vi "getHWIO_4_statusExpos.vi"(0 "Camera in":refnum<class "Camera.lvclass">, 5 "error in (no error)":errorcluster) -> (14 "Camera out":refnum<class "Camera.lvclass">, 15 "on":bool=TRUE, 16 "polarity":u16(ring)=1 items=["high level"=1, "low level"=2], 17 "signal_type":u32(ring)=1 items=["Status Busy", "Status Expos", "Status Line", "Status Armed"], 18 "signal_timing":u32(ring) items=["undefined", "first line", "global", "last line", "all lines"], 19 "error out":errorcluster)   [LabVIEW 2019, in "Camera.lvclass"]
doc: "Gets polarity, status (enabled / disabled), fuction (exposure or line) and signal timing (first line, last line, all lines, global) for the HWIO 4 status expose signal. Generates an error if camera is recording or if HWIO configuration is not supported. Signal timing is ignored if the signal function is not Status Expose."
uses:
  Camera.lvclass
  pco.sdk/TimingControl/TimingControl.lvlib
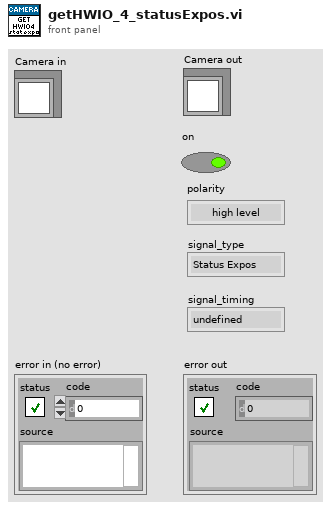
[diagram p1: front panel]
types:
  T1 = cluster{"wSignalNum":u16, "wEnabled":u16, "wType":u16, "wPolarity":u16, "wFilterSetting":u16, "wSelected":u16, "dwParameter":u32[], "dwSignalFunctionality":u32[]}
  T2 = cluster{"strSignalName":string[], "wSignalDefinitions":u16, "wSignalTypes":u16, "wSignalPolarity":u16, "wSignalFilter":u16}
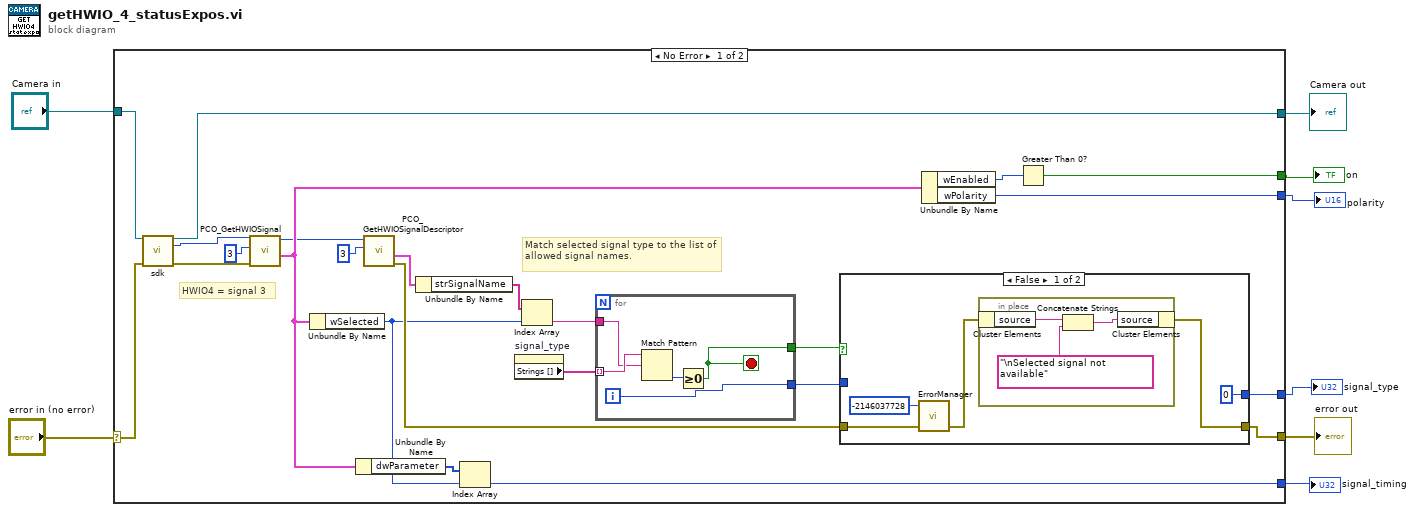
[diagram p0: block diagram]
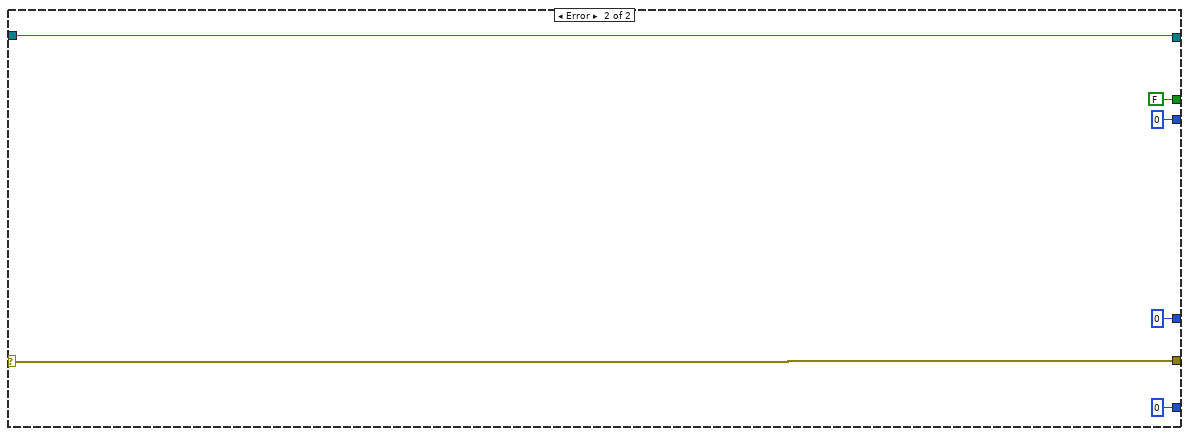
[diagram p3: hidden frame]
diagram:
  n1 = case shown="No Error" "error in (no error)" {
    selector: "error in (no error)" -> [w32 w53]
    tunnel: [w17 w53] -> w7
    tunnel: "Camera in" -> [w31 w52]
    tunnel: [w16 w52] -> w5
    tunnel: [w13 FALSE] -> w4
    tunnel: [w12 u16 0 ("wPolarity")] -> w3
    tunnel: [w11 0] -> w2
    tunnel: [w10 u32 0] -> w1
    frame No Error {
      # "Match selected signal type to the list of allowed signal names."
      # "HWIO4 = signal 3"
      n2 = call-dynamic "sdk.vi"("Camera in"=w31, "error in (no error)"=w32) -> ("Camera out"=w16:refnum<class "Camera.lvclass">, "sdk"=w30:u64, "error out"=w27:errorcluster)  [unwired: 11 in]
      n3 = call "PCO_GetHWIOSignal.vi"("error in (no error)"=w27, "wSignalNum"=u16 3, "ph"=w30) -> ("strSignal"=w15:T1, "ph out"=w9:u64)  [unwired: 5 in, 2 out]
      n4 = Unbundle By Name(w15) -> ("wSelected"=w18:u16)
      n5 = Unbundle By Name(w15) -> ("dwParameter"=w19:u32[])
      n6 = call "PCO_GetHWIOSignalDescriptor.vi"("wSignalNum"=u16 3, "ph"=w9) -> ("error out"=w22:errorcluster, "strSignalDesc"=w23:T2)  [unwired: 6 in, 2 out]
      n7 = Unbundle By Name(w23) -> ("strSignalName"=w26:string[])
      n8 = Index Array(array=w19, index=w18) -> (element=w10:u32)
      n9 = property on="signal_type" class="Ring (strict)"() -> ("Strings []"=w24:string[])  [unwired: 2 in, 2 out]
      n10 = Index Array(array=w26, index=w18) -> (element=w25:string)
      n11 = for {
        tunnel: [w46] -> w21
        tunnel: [w45] -> w20
        tunnel: w24 -> [w44] mode=indexing
        tunnel: w25 -> [w43]
        i -> [w46]
        stop <- w45 stop-if-true
        n12 = Match Pattern(string=w44, regular expression=w43) -> (offset past match=w47:i32)  [unwired: 1 in, 3 out]
        n13 = Greater Or Equal To 0?(x=w47) -> (x >= 0?=w45:bool)
      }
      n14 = case shown="False" w20 {
        tunnel: w22 -> [w37 w42]
        tunnel: [w34 w42] -> w17
        tunnel: w21 -> [_ w41]
        tunnel: [0 w41] -> w11
        frame False {
          n15 = call "ErrorManager.vi"("error in (no error)"=w37, "error code"=-2146037728) -> ("error out"=w35:errorcluster)  [unwired: 2 in, 1 out]
          n16 = in-place {
            n17 = in-place-cluster #1(w35) -> ("source"=w40:string)
            n18 = Concatenate Strings(w40, "\nSelected signal not available" ("string")) -> (w39:string)
            n19 = in-place-cluster #1("source"=w39) -> (w34:errorcluster)
          }
        }
        frame True {
        }
      }
      n20 = Unbundle By Name(w15) -> ("wEnabled"=w14:u16, "wPolarity"=w12:u16)
      n21 = Greater Than 0?(x=w14) -> (x > 0?=w13:bool)
    }
    frame Error {
    }
  }
  "Camera out" <- w5
  "error out" <- w7
  "signal_type" <- w2
  "signal_timing" <- w1
  "on" <- w4
  "polarity" <- w3
